vi "Page_AddAnalysis.vi"(8 "error in (no error)":errorcluster, 11 "Configuration Paths":T1) -> (0 "error out":errorcluster, 3 "Configuration Paths out":T1)   [LabVIEW 2010]
uses:
  Config cluster.ctl
panel:
  in  "Delete":bool
  in  "Selected analysis scripts":i32(listbox)
  in  "Add Script":bool
  out "Test Procedure":string
  in  "Cancel Button":bool
  in  "OK Button":bool
  in  "Analysis Script(source)":i32[](listbox)
  # "1) Select the analysis script(s) to be used:"
  # "Available Analsys Scripts"
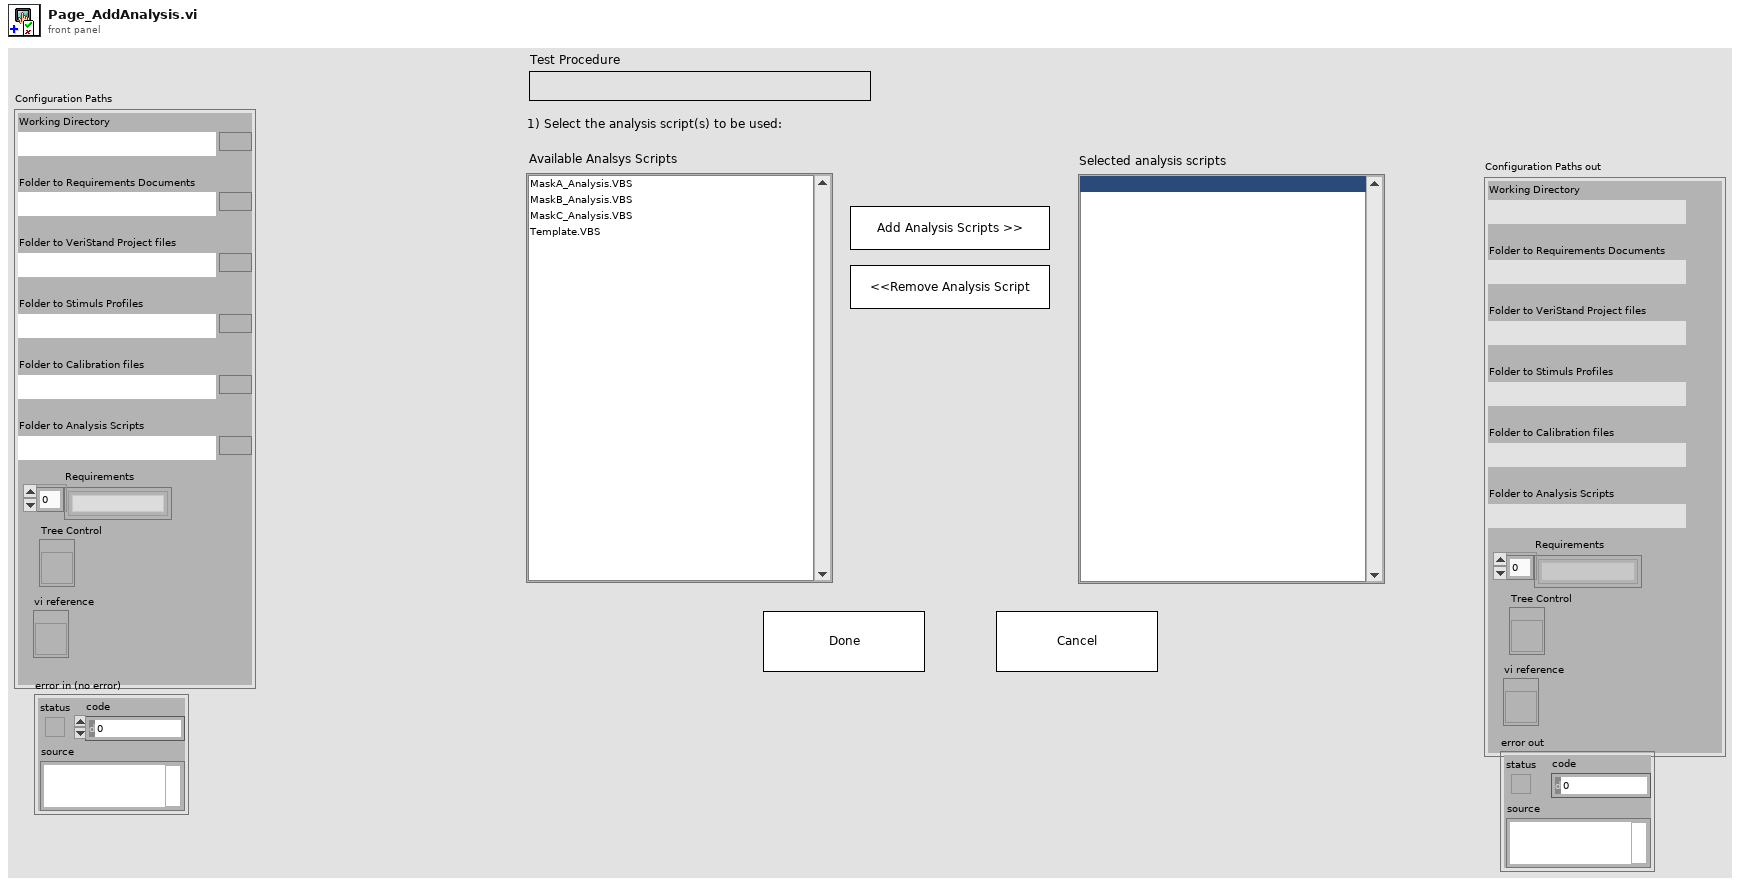
[diagram p1: front panel]
types:
  T1 = typedef "Config cluster.ctl" = cluster{"Working Directory":path, "Folder to Requirements Documents":path, "Folder to VeriStand Project files":path, "Folder to Stimuls Profiles":path, "Folder to Calibration files":path, "Folder to Analysis Scripts":path, "Requirements":string[], "Tree Control":refnum<vi>, "vi reference":refnum<vi>}
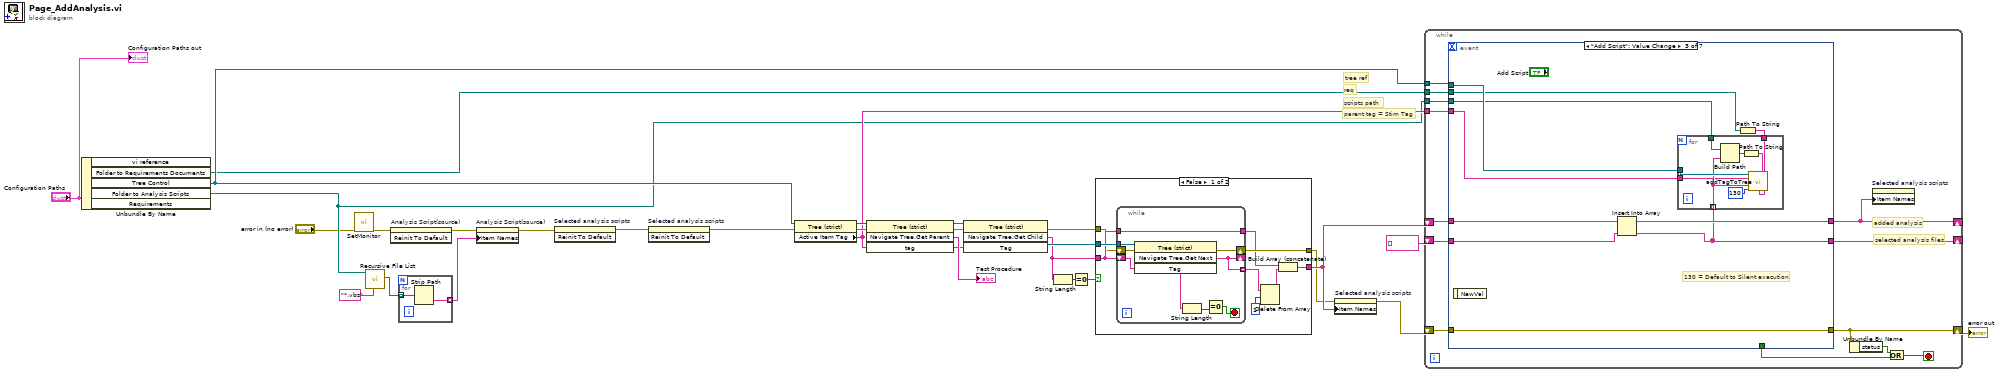
[diagram p0: block diagram]
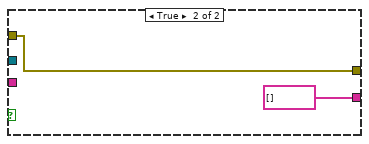
[diagram p2: hidden frame]
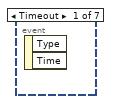
[diagram p3: hidden frame]
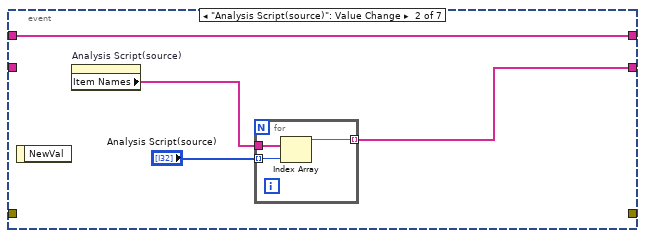
[diagram p4: hidden frame]
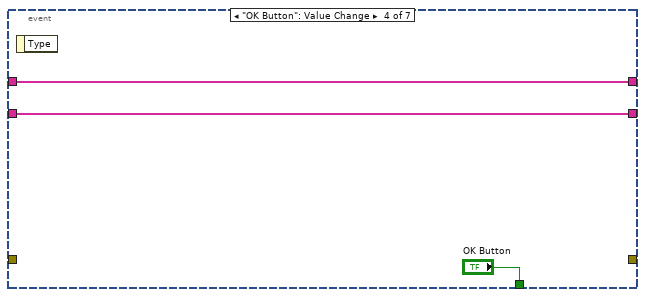
[diagram p5: hidden frame]
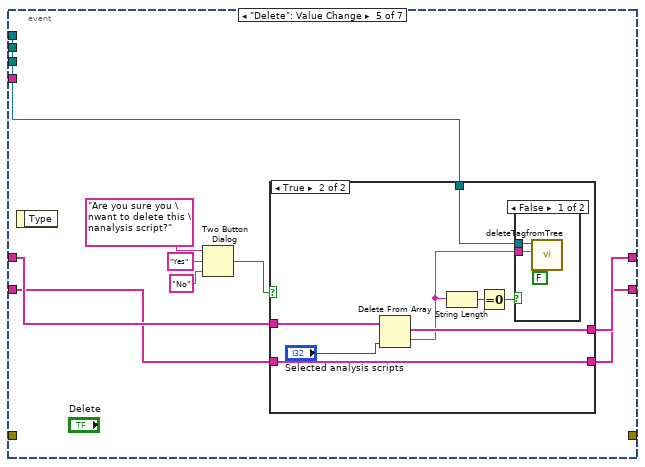
[diagram p6: hidden frame]
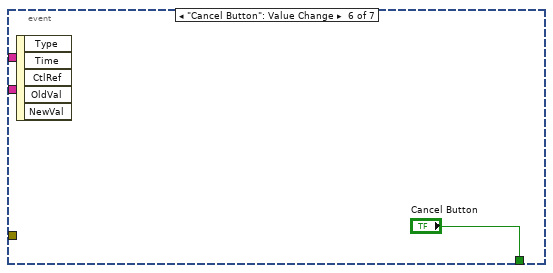
[diagram p9: hidden frame]
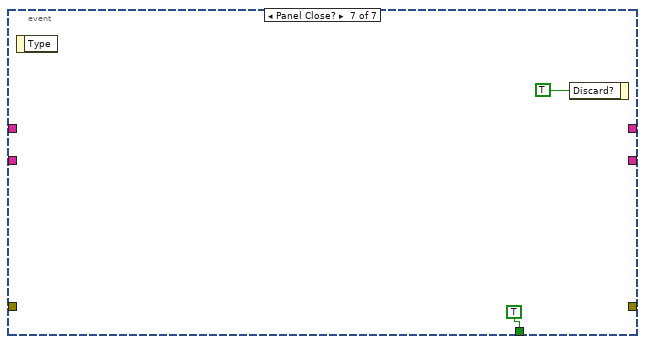
[diagram p10: hidden frame]
diagram:
  # "parent tag = Stim Tag"
  # "req"
  # "scripts path"
  # "tree ref"
  n1 = Unbundle By Name("Configuration Paths") -> ("Folder to Requirements Documents"=w16:path, "Tree Control"=w17:refnum<vi>, "Folder to Analysis Scripts"=w4:path)  [unwired: 2 out]
  n2 = call "SetMonitor.vi"("error in (no error)"="error in (no error)") -> ("error out"=w2:errorcluster)  [unwired: 9 in, 1 out]
  n3 = call <vilib>:"Recursive File List.vi"("pattern"="*.vbs", "Folder Path"=w4) -> ("All Files in Dir"=w21:path[])  [unwired: 5 in, 4 out]
  n4 = invoke on="Analysis Script(source)" class="LstBox (strict)" method="Reinit To Default"(error in=w2) -> (error out=w23:errorcluster)  [unwired: 2 in, 2 out]
  n5 = for {
    tunnel: w21 -> [w31] mode=indexing
    tunnel: [w30] -> w20 mode=indexing
    n6 = Strip Path(path=w31) -> (name=w30:string)  [unwired: 1 out]
  }
  n7 = property on="Analysis Script(source)" class="LstBox (strict)"(error in=w23, "Item Names"=w20) -> (error out=w19:errorcluster)  [unwired: 1 in, 1 out]
  n8 = invoke on="Selected analysis scripts" class="LstBox (strict)" method="Reinit To Default"(error in=w19) -> (error out=w29:errorcluster)  [unwired: 2 in, 2 out]
  n9 = invoke on="Selected analysis scripts" class="LstBox (strict)" method="Reinit To Default"(error in=w29) -> (error out=w3:errorcluster)  [unwired: 2 in, 2 out]
  n10 = property class="Tree (strict)"(reference=w17, error in=w3) -> (reference out=w11:refnum<vi>, error out=w10:errorcluster, "Active Item Tag"=w6:string)
  n11 = invoke class="Tree (strict)" method="Navigate Tree.Get Parent"(reference=w11, error in=w10, "tag"=w6) -> (reference out=w8:refnum<vi>, error out=w9:errorcluster, "Navigate Tree:Get Parent"=→"Test Procedure":string)  [unwired: 1 in, 1 out]
  n12 = invoke on="Invoke Node" class="Tree (strict)" method="Navigate Tree.Get Child"(reference=w8, error in=w9, "Tag"=w6) -> (reference out=w28:refnum<vi>, error out=w18:errorcluster, "Navigate Tree:Get Child"=w27:string)  [unwired: 1 in, 1 out]
  n13 = String Length(string=w27) -> (length=w26:i32)
  n14 = Equal To 0?(x=w26) -> (x = 0?=w25:bool)
  n15 = case shown="False" w25 {
    tunnel: [w40 w49] -> w15
    tunnel: w28 -> [w39 _]
    tunnel: [w36 string[] []] -> w24
    tunnel: w27 -> [w37 _]
    tunnel: w18 -> [w35 w49]
    frame False {
      n16 = while {
        shift-right: [w45] -> _
        shift-left: w37 -> [w44]
        tunnel: [w45] -> w34 mode=indexing
        tunnel: w39 -> [w43]
        tunnel: [w42] -> w38
        tunnel: w37 -> [w42]
        shift-right: [w46] -> w40
        shift-left: w35 -> [w41]
        stop <- w47 stop-if-true
        n17 = invoke on="Invoke Node" class="Tree (strict)" method="Navigate Tree.Get Next"(reference=w43, error in=w41, "Tag"=w44) -> (error out=w46:errorcluster, "Navigate Tree:Get Next Item"=w45:string)  [unwired: 1 in, 2 out]
        n18 = String Length(string=w45) -> (length=w48:i32)
        n19 = Equal To 0?(x=w48) -> (x = 0?=w47:bool)
      }
      n20 = Delete From Array(array=w34, length=1) -> (array with subset deleted=w32:string[])  [unwired: 1 in, 1 out]
      n21 = Build Array (concatenate)(w38, w32) -> (w36:string[])
    }
    frame True {
    }
  }
  n22 = property on="Selected analysis scripts" class="LstBox (strict)"(error in=w15, "Item Names"=w24) -> (error out=w14:errorcluster)  [unwired: 1 in, 1 out]
  n23 = while {
    shift-right: [w62] -> _
    shift-left: string[] [] -> [w61]
    shift-right: [w59] -> _
    shift-left: w24 -> [w60]
    tunnel: w17 -> [w58]
    tunnel: w16 -> [w57]
    tunnel: w4 -> [w63]
    shift-right: [w55] -> w13
    shift-left: w14 -> [w56]
    tunnel: w6 -> [w51]
    stop <- w52 stop-if-true
    # "added analysis"
    # "selected analysis files"
    n24 = event shown="[2] \"Add Script\": Value Change" {
      selector: _ -> [_ _ _ _ _ _ _]
      dyn-events: _ -> [_ _ _ _ _ _ _]
      timeout: _ -> [_ _ _ _ _ _ _]
      tunnel: w63 -> [_ _ w75 _ _ _ _]
      tunnel: [_ _ _ "OK Button" _ "Cancel Button" TRUE ("Cancel Button")] -> w53
      tunnel: [_ w67 w76 w89 w92 _ _] -> w62
      tunnel: w61 -> [_ _ w76 w89 w93 _ _]
      tunnel: w60 -> [_ w66 w79 w88 w99 _ _]
      tunnel: [_ w66 w77 w88 w98 _ _] -> w59
      tunnel: w58 -> [_ _ w78 _ w97 _ _]
      tunnel: w57 -> [_ _ w74 _ _ _ _]
      tunnel: w56 -> [_ _ w72 _ _ _ _]
      tunnel: [_ _ w72 _ _ _ _] -> w55
      tunnel: w51 -> [_ _ w71 _ _ _ _]
      event Timeout {
        n25 = event-data() -> ()  [unwired: 1 in, 2 out]
      }
      event "Analysis Script(source)": Value Change {
        n26 = event-data() -> ()  [unwired: 1 in, 1 out]
        n27 = property on="Analysis Script(source)" class="LstBox (strict)"() -> ("Item Names"=w64:string[])  [unwired: 2 in, 2 out]
        n28 = for {
          tunnel: [w70] -> w67 mode=indexing
          tunnel: w64 -> [w69]
          tunnel: "Analysis Script(source)" -> [w68] mode=indexing
          n29 = Index Array(array=w69, index=w68) -> (element=w70:string)
        }
      }
      event "Add Script": Value Change {
        # "130 = Default to Silent execution"
        n30 = event-data() -> ()  [unwired: 1 in, 1 out]
        n31 = Insert Into Array(array=w79, new element=w76) -> (w77:string[])  [unwired: 1 in]
        n32 = Path To String(path=w74) -> (string=w73:string)
        n33 = for {
          tunnel: w78 -> [w87]
          tunnel: w76 -> [w85] mode=indexing
          tunnel: w75 -> [w84]
          tunnel: w73 -> [w81]
          tunnel: w71 -> [w80]
          n34 = Build Path(base path=w84, name or relative path=w85) -> (appended path=w83:path)
          n35 = Path To String(path=w83) -> (string=w82:string)
          n36 = call "addTagToTree.vi"("Tree ref"=w87, "parent tag"=w80, "new tag"=w85, "Symbol"=130, "Req doc path"=w81, "Analysis script path"=w82) -> ()  [unwired: 9 in, 1 out]
        }
      }
      event "OK Button": Value Change {
        n37 = event-data() -> ()  [unwired: 1 in, 1 out]
      }
      event "Delete": Value Change {
        n38 = event-data() -> ()  [unwired: 1 in, 1 out]
        n39 = Two Button Dialog(message="Are you sure you \nwant to delete this \nanalysis script?", 1:"No" ("F button name (\"Cancel\")"), 2:"Yes" ("T button name (\"OK\")")) -> (T button?=w91:bool)
        n40 = case shown="True" w91 {
          tunnel: w99 -> [w101 w108]
          tunnel: [w101 w107] -> w98
          tunnel: w97 -> [_ w106]
          tunnel: w93 -> [w100 w105]
          tunnel: [w100 w105] -> w92
          frame False {
          }
          frame True {
            n41 = Delete From Array(array=w108, index="Selected analysis scripts") -> (deleted portion=w104:string, array with subset deleted=w107:string[])  [unwired: 1 in]
            n42 = String Length(string=w104) -> (length=w103:i32)
            n43 = Equal To 0?(x=w103) -> (x = 0?=w102:bool)
            n44 = case shown="False" w102 {
              tunnel: w106 -> [w112 _]
              tunnel: w104 -> [w110 _]
              frame False {
                n45 = call "deleteTagfromTree.vi"("Delete Children?"=FALSE, "Tag"=w110, "Tree Ref"=w112) -> ()  [unwired: 7 in, 2 out]
              }
              frame True {
              }
            }
          }
        }
      }
      event "Cancel Button": Value Change {
        n46 = event-data() -> ()  [unwired: 1 in, 5 out]
      }
      event Panel Close? {
        n47 = event-data() -> ()  [unwired: 1 in, 1 out]
        n48 = event-data("Discard?"=TRUE) -> ()  [unwired: 1 in, 1 out]
      }
    }
    n49 = Unbundle By Name(w55) -> ("status"=w54:bool)
    n50 = property on="Selected analysis scripts" class="LstBox (strict)"("Item Names"=w59) -> ()  [unwired: 2 in, 2 out]
    n51 = Or(x=w54, y=w53) -> (x .or. y?=w52:bool)
  }
  "error out" <- w13
  "Configuration Paths out" <- "Configuration Paths"
